vi "Write Control XBox Controller Layout Ref.vi"(8 "error in (no error)":errorcluster, 10 "XBox Controller Layout Ref":refnum<vi>, 11 "XboxController-V in":refnum<class "XboxController-V.lvclass">) -> (0 "error out":errorcluster, 3 "XboxController-V out":refnum<class "XboxController-V.lvclass">)   [LabVIEW 2013, in "XboxController-V.lvclass"]
uses:
  XboxController-V.lvclass
  XboxController-V.lvclass/XboxController-V.ctl
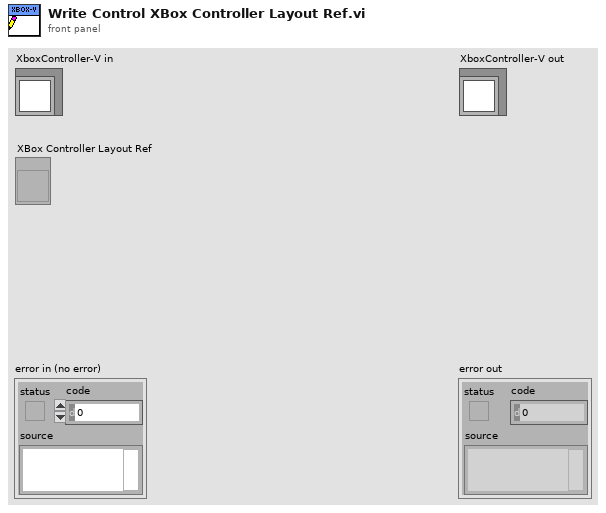
[diagram p1: front panel]
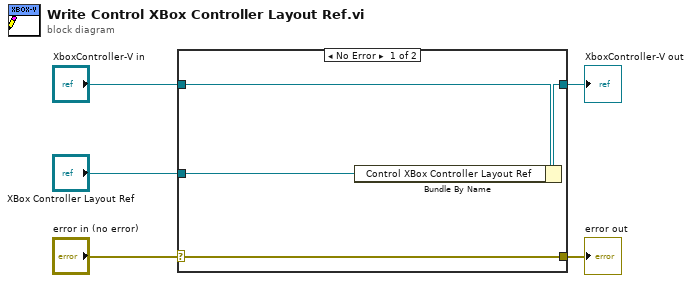
[diagram p0: block diagram]
diagram:
  n1 = case shown="No Error" "error in (no error)" {
    selector: "error in (no error)" -> [w9 w10]
    tunnel: [w9 w10] -> w4
    tunnel: [w7 w11] -> w2
    tunnel: "XboxController-V in" -> [w8 w11]
    tunnel: "XBox Controller Layout Ref" -> [w6 _]
    frame No Error {
      n2 = Bundle By Name(cluster=w8, "Control XBox Controller Layout Ref"=w6) -> (w7:refnum<class "XboxController-V.lvclass">)
    }
    frame Error {
    }
  }
  "error out" <- w4
  "XboxController-V out" <- w2
